vi "ColorEncode.vi"(0 "thresholds":T1={"1"=1.0, "2"=1.0, "3"=1.0, "4"=1.0, "5"=1.0} {"5" format="%.2f"; "4" format="%.2f"; "3" format="%.2f"; "2" format="%.2f"; "1" format="%.2f"}, 1 "midband in":dbl[][](array[numeric]), 2 "intercept in":dbl[][](array[numeric]), 3 "score in":dbl[][](array[numeric]) format="%.2f", 4 "scaled score":dbl[][](array[numeric]) format="%.2f") -> (5 "midband out":dbl[][](array[numeric]), 6 "intercept out":dbl[][](array[numeric]), 7 "scaled score out":dbl[][](array[numeric]) format="%.2f")   [LabVIEW 2022 SP3]
panel:
  out "score out":dbl[][](graph)
  # "5 is highest likelihood. If make unsuded values equal to lowest valid threshold"
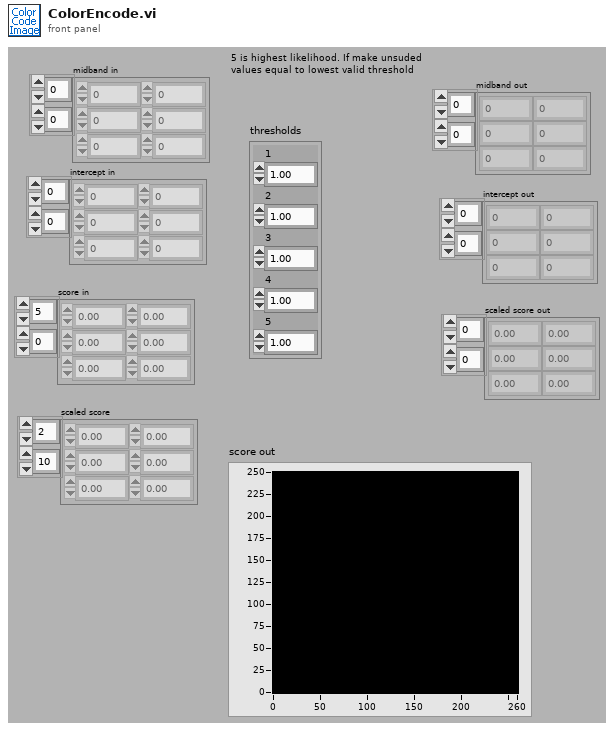
[diagram p1: front panel]
types:
  T1 = cluster{"1":dbl, "2":dbl, "3":dbl, "4":dbl, "5":dbl}
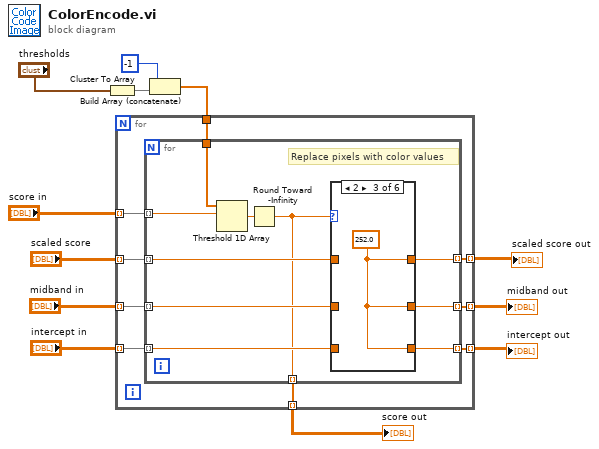
[diagram p0: block diagram]
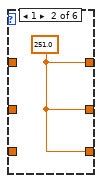
[diagram p3: hidden frame]
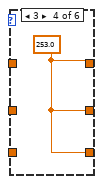
[diagram p4: hidden frame]
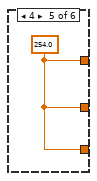
[diagram p5: hidden frame]
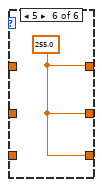
[diagram p6: hidden frame]
diagram:
  n1 = Cluster To Array(cluster="thresholds") -> (array=w5:dbl[])
  n2 = Build Array (concatenate)(-1, w5) -> (w4:dbl[])
  n3 = for {
    tunnel: "score in" -> [w21] mode=indexing
    tunnel: w4 -> [w20]
    tunnel: "midband in" -> [w19] mode=indexing
    tunnel: "intercept in" -> [w18] mode=indexing
    tunnel: [w17] -> w8 mode=indexing
    tunnel: [w16] -> w7 mode=indexing
    tunnel: [w15] -> w6 mode=indexing
    tunnel: "scaled score" -> [w14] mode=indexing
    tunnel: [w13] -> w1 mode=indexing
    n4 = for {
      tunnel: w21 -> [w25] mode=indexing
      tunnel: w20 -> [w31]
      tunnel: w19 -> [w29] mode=indexing
      tunnel: w18 -> [w28] mode=indexing
      tunnel: [w27] -> w17 mode=indexing
      tunnel: [w26] -> w16 mode=indexing
      tunnel: [w24] -> w15 mode=indexing
      tunnel: w14 -> [w23] mode=indexing
      tunnel: [w22] -> w13 mode=indexing
      # "Replace pixels with color values"
      n5 = Threshold 1D Array(2:w25, 3:w31) -> (0:w30:dbl)  [unwired: 1 out]
      n6 = Round Toward -Infinity(1:w30) -> (0:w22:dbl)
      n7 = case shown="2" w22 {
        tunnel: [w34 w35 w36 w37 w38 w39] -> w26
        tunnel: w29 -> [w34 _ _ _ _ _]
        tunnel: [w33 w35 w36 w37 w38 w39] -> w27
        tunnel: w28 -> [w33 _ _ _ _ _]
        tunnel: [w32 w35 w36 w37 w38 w39] -> w24
        tunnel: w23 -> [w32 _ _ _ _ _]
        frame 0, Default {
        }
        frame 1 {
          w35 = 251.0
        }
        frame 2 {
          w36 = 252.0
        }
        frame 3 {
          w37 = 253.0
        }
        frame 4 {
          w38 = 254.0
        }
        frame 5 {
          w39 = 255.0
        }
      }
    }
  }
  "scaled score out" <- w6
  "midband out" <- w7
  "intercept out" <- w8
  "score out" <- w1
